vi "Number of values for avg.vi"(8 "error in":errorcluster, 11 "Avg period (h)":i32) -> (0 "error out":errorcluster, 3 "Number of values for avg":dbl)   [LabVIEW 2017, in "Akwizycja.lvlib"]
uses:
  Akwizycja.lvlib
  <vilib>/Utility/config.llb/NI_LVConfig.lvlib
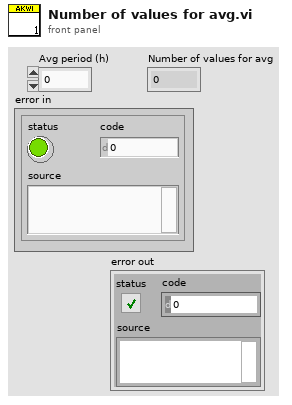
[diagram p1: front panel]
types:
  T1 = typedef "NI_LVConfig.lvlib/Config Data RefNum.ctl" = refnum<k1>
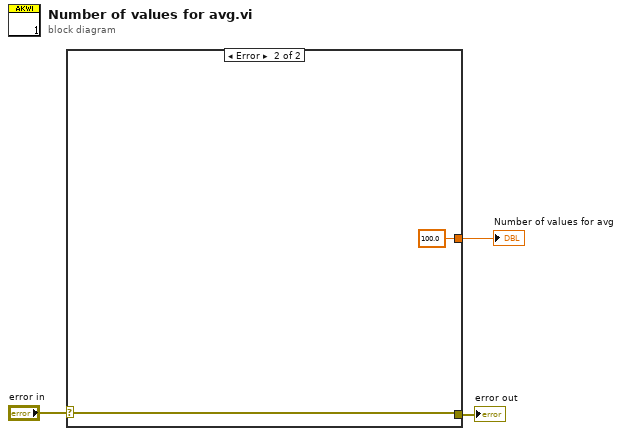
[diagram p0: block diagram]
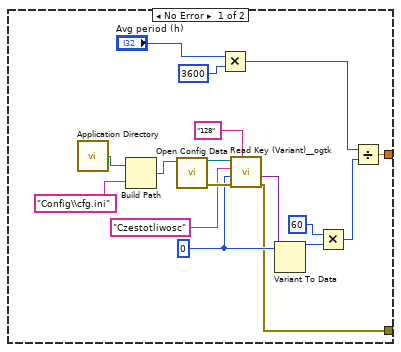
[diagram p2: hidden frame]
diagram:
  n1 = case shown="Error" "error in" {
    selector: "error in" -> [_ w22]
    tunnel: [w20 100.0] -> w3
    tunnel: [w4 w22] -> w1
    frame No Error {
      w9 = 0
      n2 = call <vilib>:"Application Directory.vi"() -> ("Application Directory"=w16:path)
      n3 = Build Path(base path=w16, name or relative path="Config\\cfg.ini") -> (appended path=w14:path)
      n4 = call <vilib>:"Open Config Data.vi"("configuration file path"=w14) -> ("error out"=w12:errorcluster, "refnum"=w13:T1)  [unwired: 8 in, 1 out]
      n5 = Multiply(x="Avg period (h)", y=3600) -> (x*y=w19:i32)
      n6 = call <userlib>:"Read Key (Variant)__ogtk.vi"("section"="128", "error in (no error)"=w12, "type"=w9, "key (optional)"="Czestotliwosc", "refnum"=w13) -> ("error out"=w4:errorcluster, "key-value"=w10:variant)  [unwired: 3 in, 2 out]
      n7 = Variant To Data(type=w9, Variant=w10) -> (data=w7:i32)  [unwired: 1 in, 1 out]
      n8 = Multiply(x=60, y=w7) -> (x*y=w5:i32)
      n9 = Divide(x=w19, y=w5) -> (x/y=w20:dbl)
    }
    frame Error {
    }
  }
  "Number of values for avg" <- w3
  "error out" <- w1
